vi "Configure Modbus Master.vi"(6 "IED Name":string, 8 "error in (no error)":errorcluster, 10 "config file refnum in":T1, 11 "IED in":refnum<class "IED.lvclass">) -> (0 "error out":errorcluster, 2 "config file refnum out":T1, 3 "IED out":refnum<class "IED.lvclass">)   [LabVIEW 2015, in "IED Actor.lvlib" / "IED.lvclass"]
uses:
  IED.lvclass
  <vilib>/Utility/config.llb/Config Data RefNum.ctl
  IED.lvclass/IED.ctl
  Controls/Comm Cluster.ctl
  <vilib>/Utility/config.llb/Read Key (String).vi
  <vilib>/Utility/config.llb/Read Key (U32).vi
  <vilib>/Utility/config.llb/NI_LVConfig.lvlib
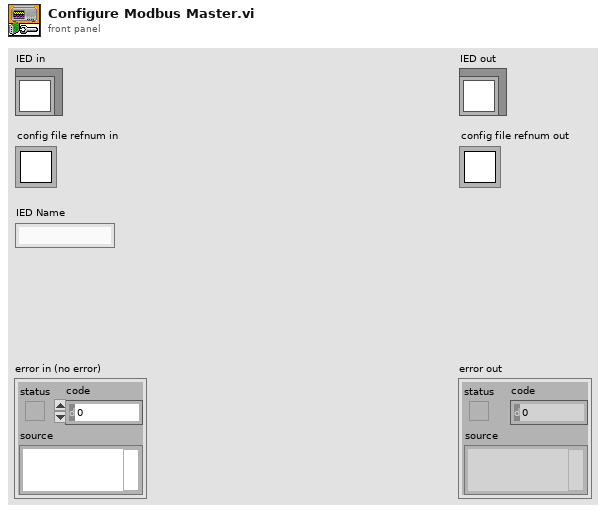
[diagram p1: front panel]
types:
  T1 = typedef "NI_LVConfig.lvlib/Config Data RefNum.ctl" = refnum<k1>
  T2 = typedef "IED Actor.lvlib/IED.lvclass/Comm Cluster.ctl" = cluster{"IP Address":string, "Port":u16}
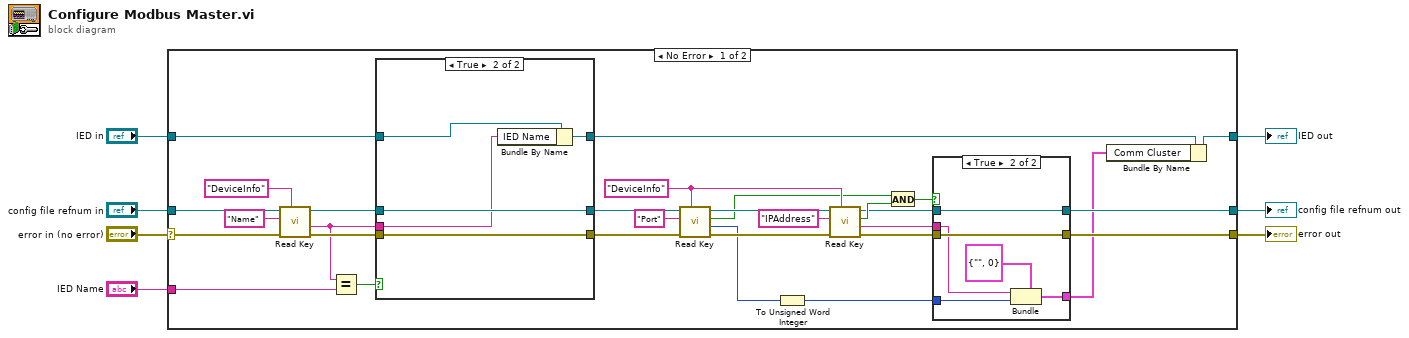
[diagram p0: block diagram]
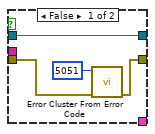
[diagram p2: hidden frame]
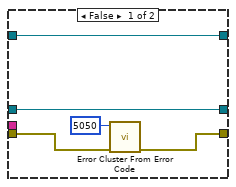
[diagram p3: hidden frame]
diagram:
  n1 = case shown="No Error" "error in (no error)" {
    selector: "error in (no error)" -> [w35 w60]
    tunnel: [w11 w60] -> w6
    tunnel: [w9 w59] -> w4
    tunnel: "IED in" -> [w29 w59]
    tunnel: "config file refnum in" -> [w37 w58]
    tunnel: [w12 w58] -> w2
    tunnel: "IED Name" -> [w33 _]
    frame No Error {
      w23 = "DeviceInfo" ("section")
      n2 = call-poly <vilib>:"Read Key.vi"("section"="DeviceInfo", "error in (no error)"=w35, "key"="Name", "refnum"=w37) -> ("error out"=w31:errorcluster, "value"=w30:string, "refnum out"=w28:T1)  [unwired: 4 in, 1 out]
      n3 = Equal?(x=w30, y=w33) -> (x = y?=w32:bool)
      n4 = case shown="True" w32 {
        tunnel: w31 -> [w52 w57]
        tunnel: w30 -> [_ w54]
        tunnel: [w51 w57] -> w25
        tunnel: w29 -> [w48 w55]
        tunnel: w28 -> [w49 w56]
        tunnel: [w49 w56] -> w26
        tunnel: [w48 w53] -> w10
        frame False {
          n5 = call <vilib>:"Error Cluster From Error Code.vi"("error in (no error)"=w52, "error code (0)"=5050) -> ("error out"=w51:errorcluster)  [unwired: 7 in]
        }
        frame True {
          n6 = Bundle By Name(cluster=w55, "IED Name"=w54) -> (w53:refnum<class "IED.lvclass">)
        }
      }
      n7 = call-poly <vilib>:"Read Key.vi"("section"=w23, "error in (no error)"=w25, "key"="Port", "refnum"=w26) -> ("error out"=w22:errorcluster, "value"=w20:u32, "found?"=w17:bool, "refnum out"=w24:T1)  [unwired: 4 in]
      n8 = To Unsigned Word Integer(number=w20) -> (unsigned 16bit integer=w15:u16)
      n9 = call-poly <vilib>:"Read Key.vi"("section"=w23, "error in (no error)"=w22, "key"="IPAddress", "refnum"=w24) -> ("error out"=w19:errorcluster, "value"=w16:string, "found?"=w18:bool, "refnum out"=w13:T1)  [unwired: 4 in]
      n10 = And(x=w17, y=w18) -> (x .and. y?=w14:bool)
      n11 = case shown="True" w14 {
        tunnel: [w38 w46] -> w11
        tunnel: w19 -> [w39 w46]
        tunnel: w16 -> [_ w44]
        tunnel: w15 -> [_ w45]
        tunnel: w13 -> [w41 w47]
        tunnel: [w41 w47] -> w12
        tunnel: [_ w42] -> w8
        frame False {
          n12 = call <vilib>:"Error Cluster From Error Code.vi"("error in (no error)"=w39, "error code (0)"=5051) -> ("error out"=w38:errorcluster)  [unwired: 7 in]
        }
        frame True {
          n13 = Bundle(cluster=T2 {"IP Address"="", "Port"=0} ("output cluster"), "IP Address"=w44, "Port"=w45) -> (w42:T2)
        }
      }
      n14 = Bundle By Name(cluster=w10, "Comm Cluster"=w8) -> (w9:refnum<class "IED.lvclass">)
    }
    frame Error {
    }
  }
  "error out" <- w6
  "IED out" <- w4
  "config file refnum out" <- w2
